vi "UTIL_ResistorStatus.vi"(8 "Status in":i16, 10 "Measure?":bool, 11 "Good!Bad":bool) -> (0 "Status out":u32, 2 "Err Num":i32)   [LabVIEW 2024]
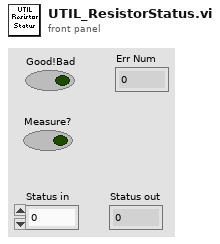
[diagram p1: front panel]
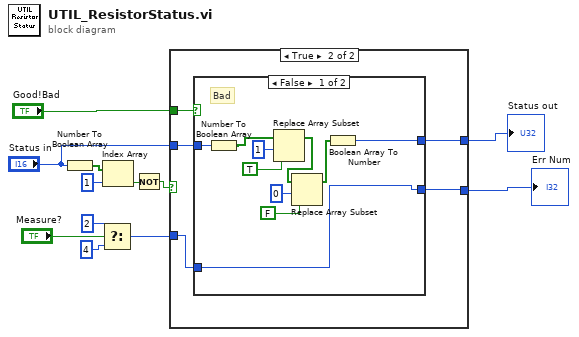
[diagram p0: block diagram]
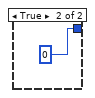
[diagram p3: hidden frame]
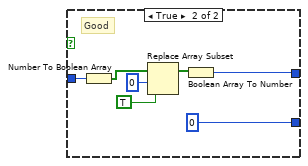
[diagram p4: hidden frame]
diagram:
  n1 = Number To Boolean Array(number="Status in") -> (Boolean array=w6:bool[])
  n2 = Select(t=2, s="Measure?", f=4) -> (s? t:f=w2:i32)
  n3 = Index Array(array=w6, index=1) -> (element=w8:bool)
  n4 = Not(x=w8) -> (.not. x?=w10:bool)
  n5 = case shown="True" w10 {
    tunnel: "Good!Bad" -> [w15 w23]
    tunnel: [w16 w22] -> w12
    tunnel: "Status in" -> [w16 w21]
    tunnel: [w14 w20] -> w5
    tunnel: w2 -> [w13 w19]
    frame False {
      # "Previously had error"
      n6 = case shown="False" w15 {
        tunnel: [w17 0] -> w14
        tunnel: w13 -> [w17 _]
        frame False {
        }
        frame True {
        }
      }
    }
    frame True {
      n7 = case shown="False" w23 {
        tunnel: w21 -> [w31 w38]
        tunnel: [w25 w35] -> w22
        tunnel: [w24 0] -> w20
        tunnel: w19 -> [w24 _]
        frame False {
          # "Bad"
          n8 = Number To Boolean Array(number=w31) -> (Boolean array=w30:bool[])
          n9 = Replace Array Subset(array=w30, new element=TRUE ("new element/subarray"), index=1) -> (w27:bool[])
          n10 = Replace Array Subset(array=w27, new element=FALSE ("new element/subarray"), index=0) -> (w26:bool[])
          n11 = Boolean Array To Number(Boolean array=w26) -> (number=w25:u32)
        }
        frame True {
          # "Good"
          n12 = Number To Boolean Array(number=w38) -> (Boolean array=w37:bool[])
          n13 = Replace Array Subset(array=w37, new element=TRUE ("new element/subarray"), index=0) -> (w36:bool[])
          n14 = Boolean Array To Number(Boolean array=w36) -> (number=w35:u32)
        }
      }
    }
  }
  "Status out" <- w12
  "Err Num" <- w5
